vi "advance array manipulation part1.vi"() -> ()   [LabVIEW 2016]
panel:
  in  "Row5":dbl
  in  "Length5":dbl
  out "Output Array52":dbl[][](array[numeric])
  out "Output Array51":dbl[][](array[numeric])
  in  "Array 5":dbl[][](array[numeric])
  in  "New Row":dbl[](array[numeric])
  in  "Row 4":dbl
  out "Out Array 4":dbl[][](array[numeric])
  in  "Array 4":dbl[][](array[numeric])
  out "Out Array 3":dbl[][](array[numeric])
  in  "New Element":dbl
  in  "Column 3":dbl
  in  "Row 3":dbl
  in  "Array 3":dbl[][](array[numeric])
  out "Output":dbl
  in  "Column2":dbl
  in  "Row2":dbl
  in  "Array 2":dbl[][](array[numeric])
  out "Size":i32[](array[numeric])
  in  "Array1":dbl[][](array[numeric])
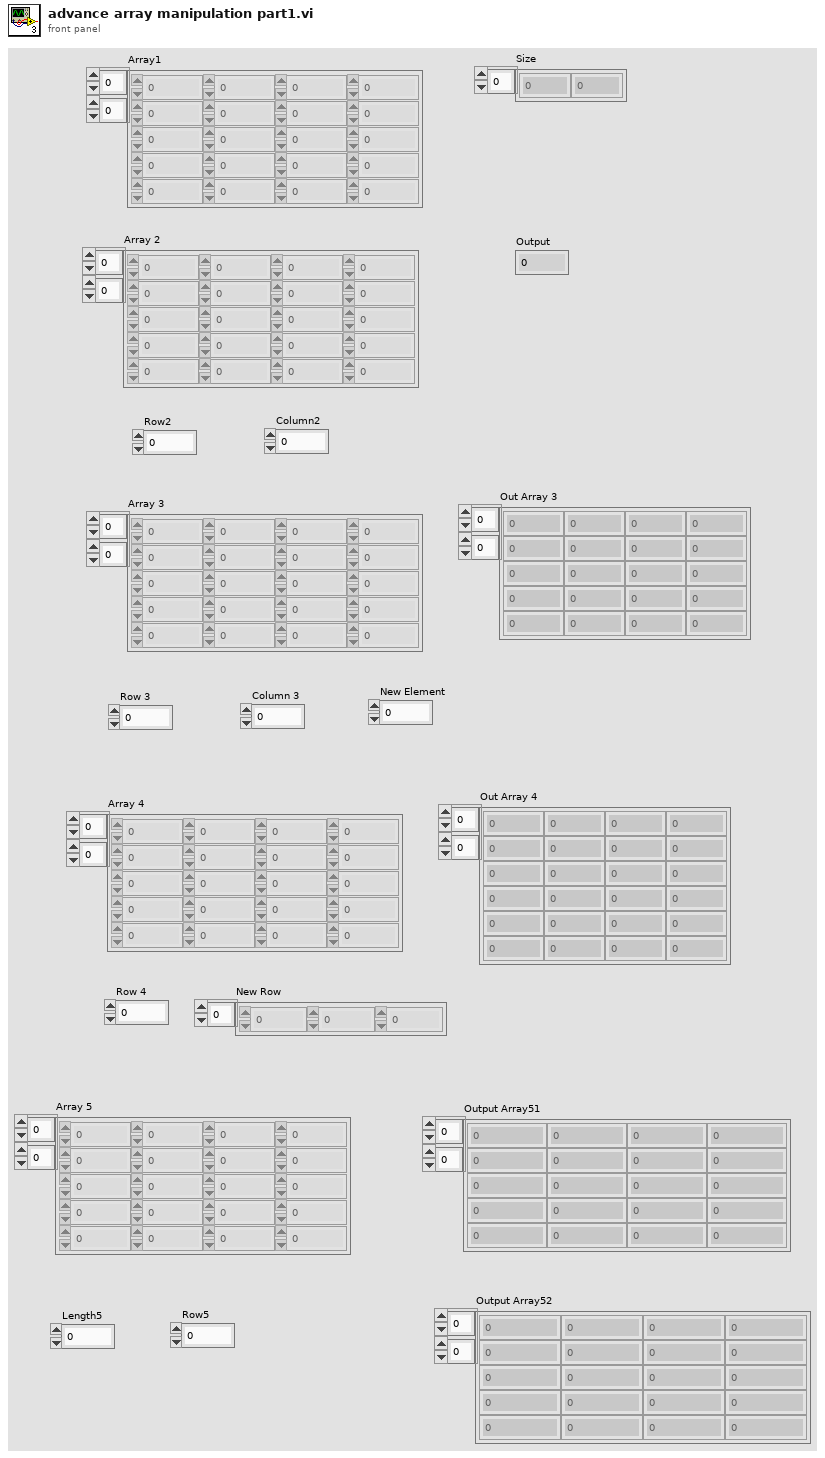
[diagram p1: front panel]
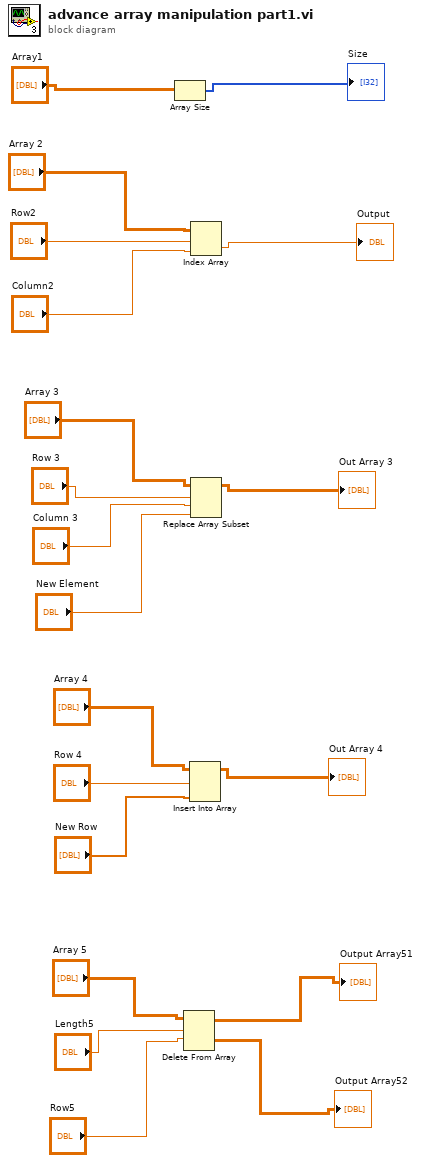
[diagram p0: block diagram]
diagram:
  n1 = Array Size(array="Array1") -> (size(s)=→"Size":i32[])
  n2 = Delete From Array "Delete From Array"(array="Array 5", length="Length5", index (row)="Row5") -> (deleted portion=→"Output Array52":dbl[][], array with subset deleted=→"Output Array51":dbl[][])  [unwired: 1 in]
  n3 = Insert Into Array "Insert Into Array"(array="Array 4", index (row)="Row 4", new element="New Row") -> (→"Out Array 4":dbl[][])  [unwired: 1 in]
  n4 = Index Array "Index Array"(array="Array 2", index (row)="Row2", index (col)="Column2") -> (element=→"Output":dbl)
  n5 = Replace Array Subset "Replace Array Subset"(array="Array 3", new element="New Element", index (row)="Row 3", index (col)="Column 3") -> (→"Out Array 3":dbl[][])
